vi "InitScope_5782.vi"(4 "RemoteConnection":refnum<class "RemoteConnection.lvclass">, 6 "Trigger":T1, 7 "Chart length":i32, 8 "error in":errorcluster, 9 "Samples Per Trigger":i32=5000000, 10 "data mode":T2, 11 "FPGA ref":T3) -> (0 "error out":errorcluster, 3 "scope params":T4)   [LabVIEW 2013]
uses:
  controls/scope_params_5782.ctl
  Utilities/Ticker/Ticker.lvclass
  Communication/Driver/RemoteConnection/RemoteConnection.lvclass
  Scope/controls/ScopeMode.ctl
  Config/FPGAref_5782.ctl
  FPGA/DataMode.ctl
  controls/5782_trigger_type.ctl
  controls/Feedforward.ctl
  FPGA/fpga_settings.ctl
  <vilib>/rvi/interface/common/niFpgaWaitOnOcc.vi
  <vilib>/Utility/error.llb/Error Cluster From Error Code.vi
  <vilib>/rvi/errors/niLvFpgaAdjustHostInterfaceError.vi
  <vilib>/rvi/FXPMathLib/FxpInterpret/XNode/nifxpmath_Interpret.xnode
  <vilib>/rvi/interface/nirviReadWriteControl/nirviReadWriteControl.xnode
  NiFpgaLv.dll
  <vilib>/rvi/interface/Simulation/niFpgaSimulationCallBeginRW.vi
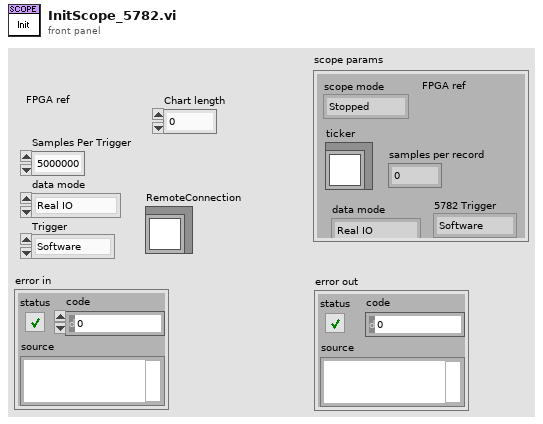
[diagram p1: front panel]
types:
  T1 = typedef "5782_trigger_type.ctl" = enum16{"Software", "Trigger input"}
  T2 = typedef "DataMode.ctl" = enum16{"Real IO", "Simulated"}
  T3 = typedef "FPGAref_5782.ctl" = refnum<k20>
  T4 = typedef "scope_params_5782.ctl" = cluster{"scope mode":T5, "ticker":refnum<class "Ticker.lvclass">, "samples per record":i32, "FPGA ref":T3, "data mode":T2, "5782 Trigger":T1, "Chart length":i32, "RemoteConnection":refnum<class "RemoteConnection.lvclass">, "last phase":dbl[], "Feedforward":T6}
  T5 = typedef "ScopeMode.ctl" = enum16{"Stopped", "Single", "Running", "Continuous"}
  T6 = typedef "Feedforward.ctl" = cluster{"Beam I":dbl[], "Beam Q":dbl[], "Feedforward I":dbl[], "Feedforward Q":dbl[], "Setpoint I":dbl[], "Setpoint Q":dbl[]}
  T7 = typedef "fpga_settings.ctl" = enum16{"Feedback Enable", "New FIR coeffs", "FIR shift", "Enable filter", "Set Downsample", "Downsample", "CIC Gain", "Record length", "Trigger samples", "Quiet time", "a_am", "b_am", "Use fixed delay", "fixed sin_fi", "fixed cos_fi", "Ki*Tau", "Kp", "Kd_Tau", "Fi_start", "Fi_delta", "DC_offs 0", "DC_offs 1", "DC_offs 2", "DC_offs 3", "Ki*Tau am", "Kp am", "Kd_Tau am", "Feedback AM", "Trigger delay", "Feedback delay", "Setpoint enable", "Beam enable", "Samples to acquire"}
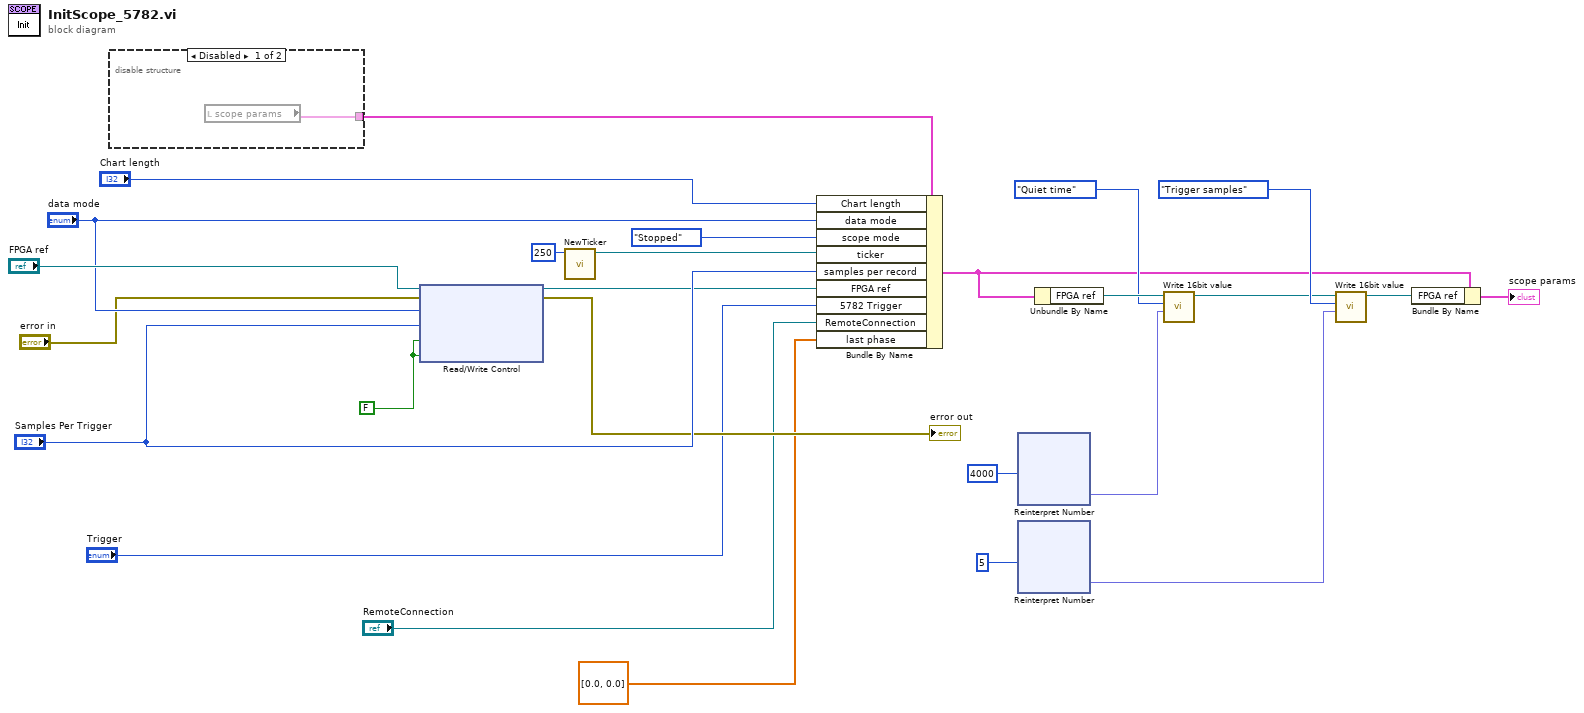
[diagram p0: block diagram]
diagram:
  w15 = FALSE
  n1 = disable-structure shown="Disabled" {
    disable-tunnel: [w27 _] -> w26
    frame Disabled {
      n2 = local read "scope params"() -> (w27:T4)
    }
    frame Enabled {
    }
  }
  n3 = xnode "Read/Write Control"("FPGA VI Reference In"="FPGA ref", "error in"="error in", "Mode"="data mode", "5782 record length"="Samples Per Trigger", "Trigger Acquisition"=w15, "Acquisition running"=w15) -> ("FPGA VI Reference Out"=w17:T3, "error out"=→"error out":errorcluster)
  n4 = call "NewTicker.vi"("Period"=u32 250) -> ("Ticker"=w23:refnum<class "Ticker.lvclass">)  [unwired: 10 in]
  n5 = Bundle By Name(cluster=w26, "Chart length"="Chart length", "data mode"="data mode", "scope mode"=ScopeMode."Stopped", "ticker"=w23, "samples per record"="Samples Per Trigger", "FPGA ref"=w17, "5782 Trigger"="Trigger", "RemoteConnection"="RemoteConnection", "last phase"=dbl[] [0.0, 0.0]) -> (w7:T4)
  n6 = xnode "Reinterpret Number"("x"=u16 4000 ("Samples to aqcuire")) -> ("y"=w3:fxp<+,16,16>)
  n7 = xnode "Reinterpret Number"("x"=u16 5 ("trigger samples")) -> ("y"=w1:fxp<+,16,16>)
  n8 = Unbundle By Name(w7) -> ("FPGA ref"=w11:T3)
  n9 = call "Write 16bit value.vi"("value"=w3, "FPGA Setting"=fpga_settings."Quiet time", "FPGA ref"=w11) -> ("FPGA ref out"=w8:T3)  [unwired: 7 in, 1 out]
  n10 = call "Write 16bit value.vi"("value"=w1, "FPGA Setting"=fpga_settings."Trigger samples", "FPGA ref"=w8) -> ("FPGA ref out"=w6:T3)  [unwired: 7 in, 1 out]
  n11 = Bundle By Name(cluster=w7, "FPGA ref"=w6) -> (→"scope params":T4)
